vi "Read value (Numeric).vi"(8 "error in (no error)":errorcluster, 9 "default value":dbl, 11 "JSON Numeric in":refnum<class "JSON Value.lvclass">) -> (0 "error out":errorcluster, 2 "value":dbl)   [LabVIEW 2016, in "JSON Value.lvclass"]
doc: "Returns the value of a JSON Numeric"
uses:
  JSON Value.lvclass
  JSON Value.lvclass/JSON Value.ctl
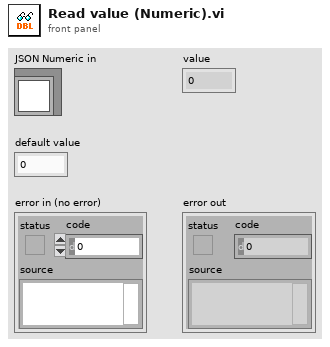
[diagram p1: front panel]
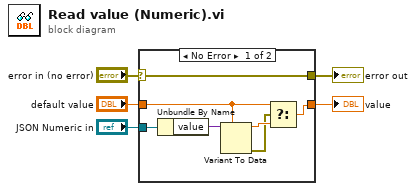
[diagram p0: block diagram]
diagram:
  n1 = case shown="No Error" "error in (no error)" {
    selector: "error in (no error)" -> [w12 w14]
    tunnel: [w12 w14] -> w4
    tunnel: "JSON Numeric in" -> [w11 _]
    tunnel: [w6 w13] -> w2
    tunnel: "default value" -> [w8 w13]
    frame No Error {
      n2 = Unbundle By Name(w11) -> ("value"=w10:variant)
      n3 = Variant To Data(type=w8, Variant=w10) -> (data=w9:dbl, error out=w7:errorcluster)  [unwired: 1 in]
      n4 = Select(t=w8, s=w7, f=w9) -> (s? t:f=w6:dbl)
    }
    frame Error {
    }
  }
  "error out" <- w4
  "value" <- w2
